vi "WebSocket Stats VIG.vi"(7 "Name":string, 8 "error in (no error)":errorcluster, 9 "RX?":bool, 10 "Length":i32, 11 "mode":T1) -> (0 "error out":errorcluster, 4 "TX Stats":variant, 6 "RX Stats":variant)   [LabVIEW 2017]
uses:
  WebSocket Stats VIG Mode.ctl
  WebSocket Stats.ctl
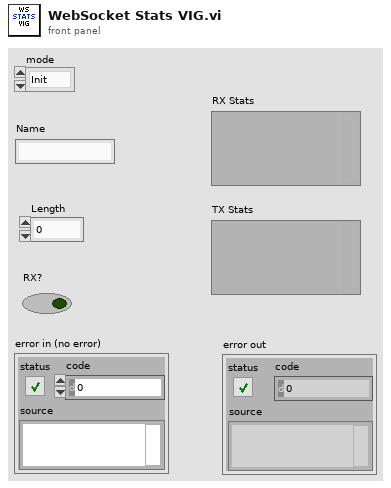
[diagram p1: front panel]
types:
  T1 = typedef "WebSocket Stats VIG Mode.ctl" = enum16{"Init", "Set", "Update", "Get All"}
  T2 = typedef "WebSocket Stats.ctl" = cluster{"T0":timestamp, "Tlast":timestamp, "Bytes":i32, "Packets":i32}
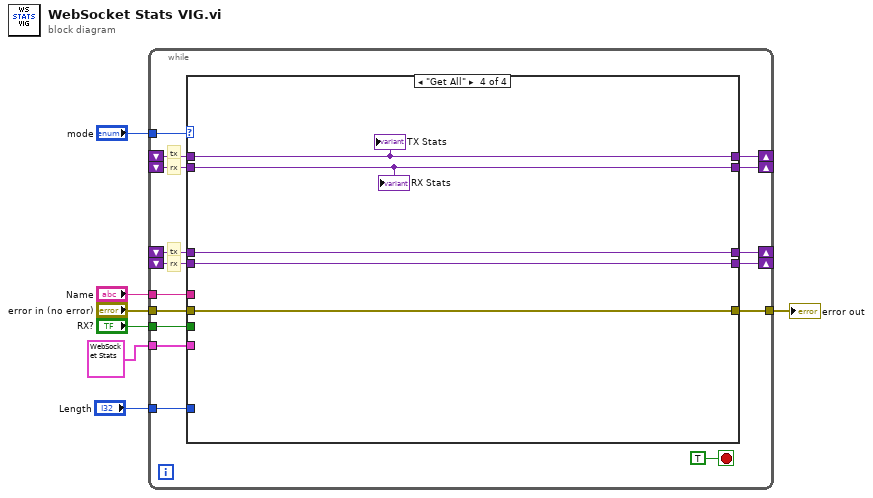
[diagram p0: block diagram]
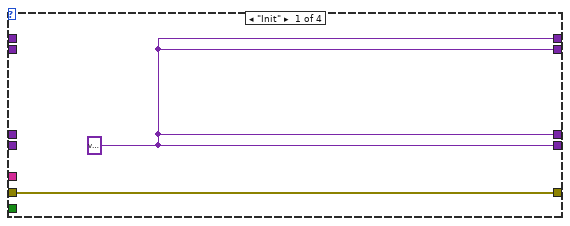
[diagram p2: hidden frame]
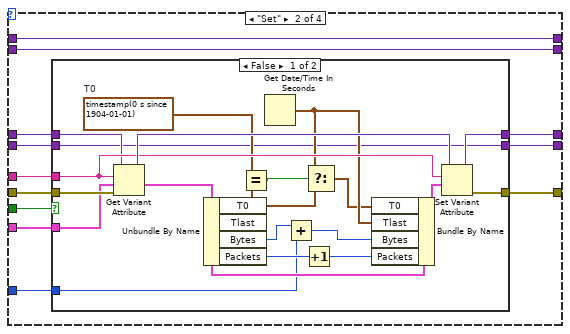
[diagram p3: hidden frame]
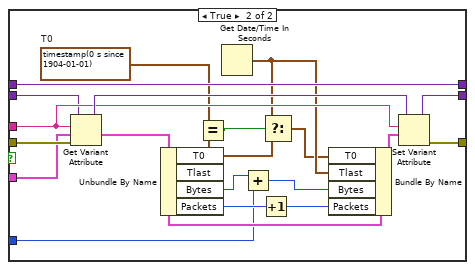
[diagram p4: hidden frame]
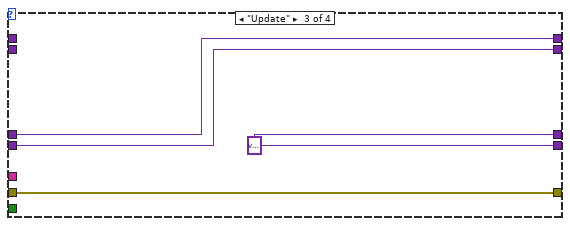
[diagram p5: hidden frame]
diagram:
  n1 = while {
    tunnel: "error in (no error)" -> [w20]
    tunnel: [w18] -> w6
    shift-right: [w19] -> _
    shift-left: _ -> [w21]
    tunnel: "mode" -> [w22]
    tunnel: "Name" -> [w17]
    tunnel: "Length" -> [w16]
    shift-right: [w15] -> _
    shift-left: _ -> [w14]
    shift-right: [w12] -> _
    shift-left: _ -> [w13]
    shift-right: [w11] -> _
    shift-left: _ -> [w10]
    tunnel: "RX?" -> [w9]
    tunnel: T2 {"T0"=timestamp(0 s since 1904-01-01), "Tlast"=timestamp(0 s since 1904-01-01), "Bytes"=0, "Packets"=0} -> [w8]
    stop <- TRUE stop-if-true
    # "tx"
    # "rx"
    # "tx"
    # "rx"
    n2 = case shown="\"Get All\"" w22 {
      tunnel: w21 -> [_ w28 w80 w85]
      tunnel: w20 -> [w25 w37 w81 w86]
      tunnel: [w24 w27 w79 w85] -> w19
      tunnel: [w25 w34 w81 w86] -> w18
      tunnel: w17 -> [_ w35 _ _]
      tunnel: w16 -> [_ w36 _ _]
      tunnel: [w24 w33 w80 w82] -> w15
      tunnel: w14 -> [_ w33 _ w82]
      tunnel: [w24 w32 w78 w83] -> w12
      tunnel: w13 -> [_ w32 _ w83]
      tunnel: w10 -> [_ w30 w78 w84]
      tunnel: [w24 w29 w79 w84] -> w11
      tunnel: w9 -> [_ w31 _ _]
      tunnel: w8 -> [_ w26 _ _]
      frame "Init" {
        w24 = variant
      }
      frame "Set" {
        n3 = case shown="False" w31 {
          tunnel: w37 -> [w57 w77]
          tunnel: w36 -> [w42 w59]
          tunnel: w35 -> [w55 w75]
          tunnel: [w54 w74] -> w34
          tunnel: w30 -> [w39 w72]
          tunnel: [w40 w72] -> w29
          tunnel: w28 -> [w38 w71]
          tunnel: [w38 w73] -> w27
          tunnel: w26 -> [w53 w70]
          frame False {
            w47 = timestamp(0 s since 1904-01-01)  # T0
            n4 = Get Variant Attribute(Variant=w39, name=w55, default value (empty Variant)=w53, error in=w57) -> (duplicate Variant=w56:variant, value=w52:T2)  [unwired: 2 out]
            n5 = Unbundle By Name(w52) -> ("T0"=w45:timestamp, "Bytes"=w43:i32, "Packets"=w50:i32)  [unwired: 1 out]
            n6 = Equal?(x=w47, y=w45) -> (x = y?=w48:bool)
            n7 = Get Date/Time In Seconds() -> (seconds since 1Jan1904=w46:timestamp)
            n8 = Add(x=w43, y=w42) -> (x+y=w41:i32)
            n9 = Increment(x=w50) -> (x+1=w49:i32)
            n10 = Select(t=w46, s=w48, f=w45) -> (s? t:f=w44:timestamp)
            n11 = Bundle By Name(cluster=w52, "T0"=w44, "Tlast"=w46, "Bytes"=w41, "Packets"=w49) -> (w51:T2)
            n12 = Set Variant Attribute(Variant=w56, name=w55, value=w51) -> (Variant out=w40:variant, error out=w54:errorcluster)  [unwired: 1 in, 1 out]
          }
          frame True {
            w64 = timestamp(0 s since 1904-01-01)  # T0
            n13 = Get Variant Attribute(Variant=w71, name=w75, default value (empty Variant)=w70, error in=w77) -> (duplicate Variant=w76:variant, value=w69:T2)  [unwired: 2 out]
            n14 = Unbundle By Name(w69) -> ("T0"=w62:timestamp, "Bytes"=w60:i32, "Packets"=w67:i32)  [unwired: 1 out]
            n15 = Equal?(x=w64, y=w62) -> (x = y?=w65:bool)
            n16 = Get Date/Time In Seconds() -> (seconds since 1Jan1904=w63:timestamp)
            n17 = Add(x=w60, y=w59) -> (x+y=w58:i32)
            n18 = Increment(x=w67) -> (x+1=w66:i32)
            n19 = Select(t=w63, s=w65, f=w62) -> (s? t:f=w61:timestamp)
            n20 = Bundle By Name(cluster=w69, "T0"=w61, "Tlast"=w63, "Bytes"=w58, "Packets"=w66) -> (w68:T2)
            n21 = Set Variant Attribute(Variant=w76, name=w75, value=w68) -> (Variant out=w73:variant, error out=w74:errorcluster)  [unwired: 1 in, 1 out]
          }
        }
      }
      frame "Update" {
        w79 = variant
      }
      frame "Get All" {
        "TX Stats" <- w83
        "RX Stats" <- w82
      }
    }
  }
  "error out" <- w6
